vi "Create User Buffer.vi"(0 "VISA resource name":refnum<visa-resource-name>, 5 "Buffer Name":string="myBuffer", 7 "Buffer Size":i32=10 min=10 step=1, 9 "Buffer Style (1: Standard)":i32(ring)=1 items=["Compact", "Standard", "Full", "Writable", "Full Writable"], 11 "error in (no error)":errorcluster) -> (4 "VISA resource name out":refnum<visa-resource-name>, 15 "error out":errorcluster)   [LabVIEW 2021, in "Keithley DMM7510.lvlib"]
doc: "This VI creates a user-defined reading buffer.\nYou cannot assign user-defined reading buffers the same name as an existing buffer, including the default buffers (defbuffer1 and defbuffer2)."
uses:
  Keithley DMM7510.lvlib
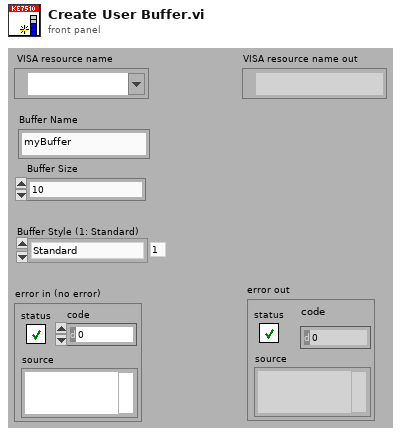
[diagram p1: front panel]
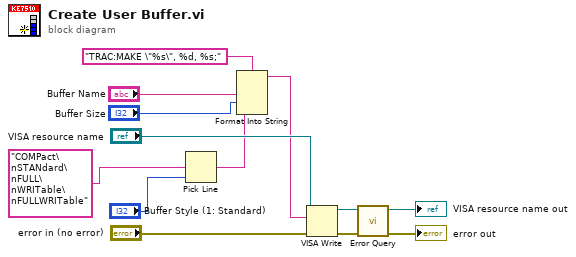
[diagram p0: block diagram]
diagram:
  n1 = Pick Line(multi-line string="COMPact\nSTANdard\nFULL\nWRITable\nFULLWRITable", line index="Buffer Style (1: Standard)") -> (output string=w1:string)  [unwired: 1 in]
  n2 = Format Into String(format string="TRAC:MAKE \"%s\", %d, %s;" ("Read Measurement"), "Buffer Name", "Buffer Size", w1) -> (resulting string=w4:string)  [unwired: 2 in, 1 out]
  n3 = VISA Write(VISA resource name="VISA resource name", write buffer=w4, error in (no error)="error in (no error)") -> (VISA resource name out=w9:refnum<visa-resource-name>, error out=w8:errorcluster)  [unwired: 1 out]
  n4 = call "Error Query.vi"("error in (no error)"=w8, "VISA resource name"=w9) -> ("error out"=→"error out":errorcluster, "VISA resource name out"=→"VISA resource name out":refnum<visa-resource-name>)  [unwired: 8 out]
